vi "Create Group Cluster.vi"(2 "Groups & Tags":cluster{string[], T1[]}[](array[cluster]), 3 "Alarm Type":string) -> (0 "CVT Groups":T3[](array[typedef]), 1 "CVT Tags":T1[](array[typedef]))   [LabVIEW 2013]
uses:
  <vilib>/NI/Current Value Table/Type Defs/Tag Grouping set.ctl
  <vilib>/NI/Current Value Table/Type Defs/Single Tag.ctl
  <vilib>/NI/Current Value Table/Type Defs/Data Types.ctl
  <vilib>/NI/Current Value Table/Current Value Table.lvlib
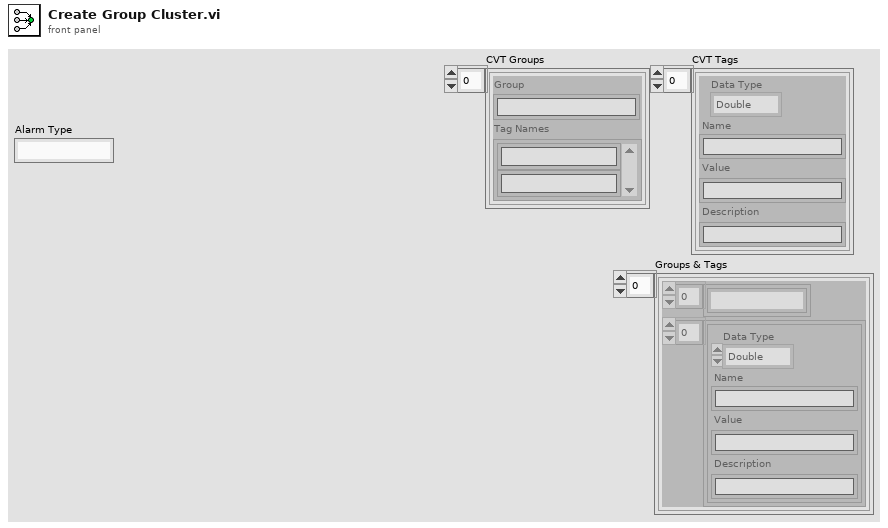
[diagram p1: front panel]
types:
  T1 = typedef "Current Value Table.lvlib/Single Tag.ctl" = cluster{"Data Type":T2, "Name":string, "Value":string, "Description":string}
  T2 = typedef "Current Value Table.lvlib/Data Types.ctl" = enum16{"Double", "Single", "I64", "I32", "I16", "I8", "U64", "U32", "U16", "U8", "String", "Boolean", "Array of U8", "Array of U16", "Array of U32", "Array of U64", "Array of I64", "Array of I32", "Array of I16", "Array of I8", "Array of Double", "Array of Single", "Array of Boolean", "Array of String"}
  T3 = typedef "Current Value Table.lvlib/Tag Grouping set.ctl" = cluster{"Group":string, "Tag Names":string[]}
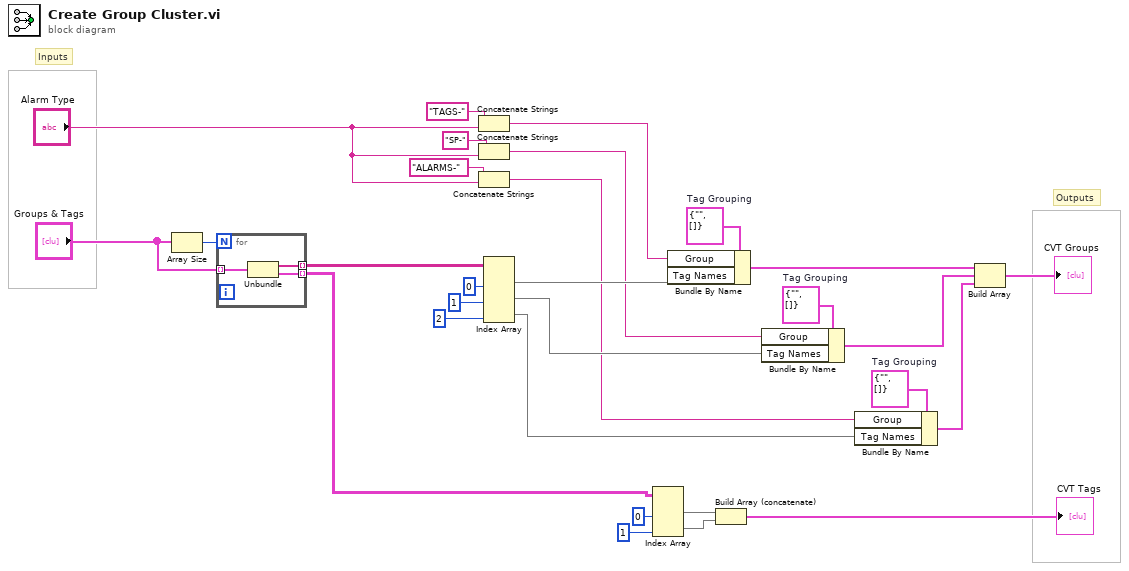
[diagram p0: block diagram]
diagram:
  w20 = T3 {"Group"="", "Tag Names"=[]}  # Tag Grouping
  w21 = T3 {"Group"="", "Tag Names"=[]}  # Tag Grouping
  w22 = T3 {"Group"="", "Tag Names"=[]}  # Tag Grouping
  # "Inputs"
  # "Outputs"
  n1 = Array Size(array="Groups & Tags") -> (size(s)=w4:i32)
  n2 = for {
    N: w4 -> [_]
    tunnel: "Groups & Tags" -> [w32] mode=indexing
    tunnel: [w31] -> w1 mode=indexing
    tunnel: [w30] -> w2 mode=indexing
    n3 = Unbundle(w32) -> (w31:string[], w30:T1[])
  }
  n4 = Concatenate Strings("TAGS-" ("string"), "Alarm Type") -> (w12:string)
  n5 = Concatenate Strings("SP-" ("string"), "Alarm Type") -> (w11:string)
  n6 = Concatenate Strings("ALARMS-" ("string"), "Alarm Type") -> (w10:string)
  n7 = Index Array(array=w1, index (col) #1=0 ("index (row)"), index (col) #2=1 ("index (row)"), index (col) #3=2 ("index (row)")) -> (element #1=w28:string[], element #2=w27:string[], element #3=w26:string[])  [unwired: 3 in]
  n8 = Index Array(array=w2, index (col) #1=0 ("index (row)"), index (col) #2=1 ("index (row)")) -> (element #1=w7:T1[], element #2=w6:T1[])  [unwired: 2 in]
  n9 = Bundle By Name(cluster=w22, "Group"=w12, "Tag Names"=w28) -> (w25:T3)
  n10 = Build Array (concatenate)(w7, w6) -> (→"CVT Tags":T1[])
  n11 = Bundle By Name(cluster=w21, "Group"=w11, "Tag Names"=w27) -> (w24:T3)
  n12 = Bundle By Name(cluster=w20, "Group"=w10, "Tag Names"=w26) -> (w23:T3)
  n13 = Build Array(w25, w24, w23) -> (→"CVT Groups":T3[])
